vi "Configure HSDIO for Dynamic Waveform.vi"(0 "Semiconductor Module Context":T1, 1 "high level (1.8 volts)":dbl=3.3 format="%.2f", 2 "low level (0.00 volts)":dbl format="%.2f", 3 "Sample Clock Rate":dbl=104000000.0 format="%#_6p", 5 "All Pins":string[](array[string])=["CLK", "SDA", "SETID", "VIO", "HV"], 11 "error in (no error)":errorcluster) -> (15 "error out":errorcluster)   [LabVIEW 2013]
uses:
  <vilib>/NI_TestStand_SemiconductorModule/NI_TestStand_Semiconductor_Module.lvlibp/PinMap/General/SemiconductorModuleContext.ctl
  <vilib>/NI_TestStand_SemiconductorModule/NI_TestStand_Semiconductor_Module.lvlibp/PinMap/General/NIInstrumentTypeIDs.ctl
  <instrlib>/niHSDIO/niHSDIO.llb/niHSDIO_ctl Sample Clock Source Values (ComboBox).ctl
  <instrlib>/niHSDIO/niHSDIO.llb/niHSDIO_ctl Generation Mode Values (Ring).ctl
  <instrlib>/niHSDIO/niHSDIO.llb/niHSDIO_ctl Voltage Logic Family Values (Ring).ctl
  <vilib>/NI_TestStand_SemiconductorModule/NI_TestStand_Semiconductor_Module.lvlibp/PinMap/HSDIO/PinsToNIHSDIOSessions.vi
  <instrlib>/niHSDIO/niHSDIO.llb/niHSDIO Configure Data Voltage Logic Family.vi
  <instrlib>/niHSDIO/niHSDIO.llb/niHSDIO Configure Initial State (U32).vi
  <instrlib>/niHSDIO/niHSDIO.llb/niHSDIO Configure Idle State (U32).vi
  <instrlib>/niHSDIO/niHSDIO.llb/niHSDIO Configure Digital Edge Start Trigger.vi
  <vilib>/NI_TestStand_SemiconductorModule/NI_TestStand_Semiconductor_Module.lvlibp
panel:
  in  "RTD Compensation Value":i32=1 min=0 max=29
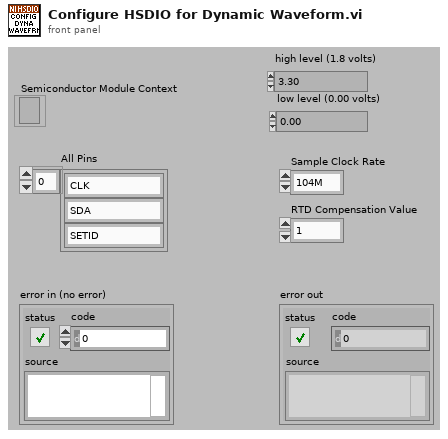
[diagram p1: front panel]
types:
  T1 = typedef "NI_TestStand_Semiconductor_Module.lvlibp/SemiconductorModuleContext.ctl" = refnum<k7>
  T2 = typedef "NI_TestStand_Semiconductor_Module.lvlibp/NIInstrumentTypeIDs.ctl" = string
  T3 = typedef "niHSDIO_ctl Voltage Logic Family Values (Ring).ctl" = i32
  T4 = typedef "niHSDIO_ctl Generation Mode Values (Ring).ctl" = i32
  T5 = typedef "niHSDIO_ctl Sample Clock Source Values (ComboBox).ctl" = string
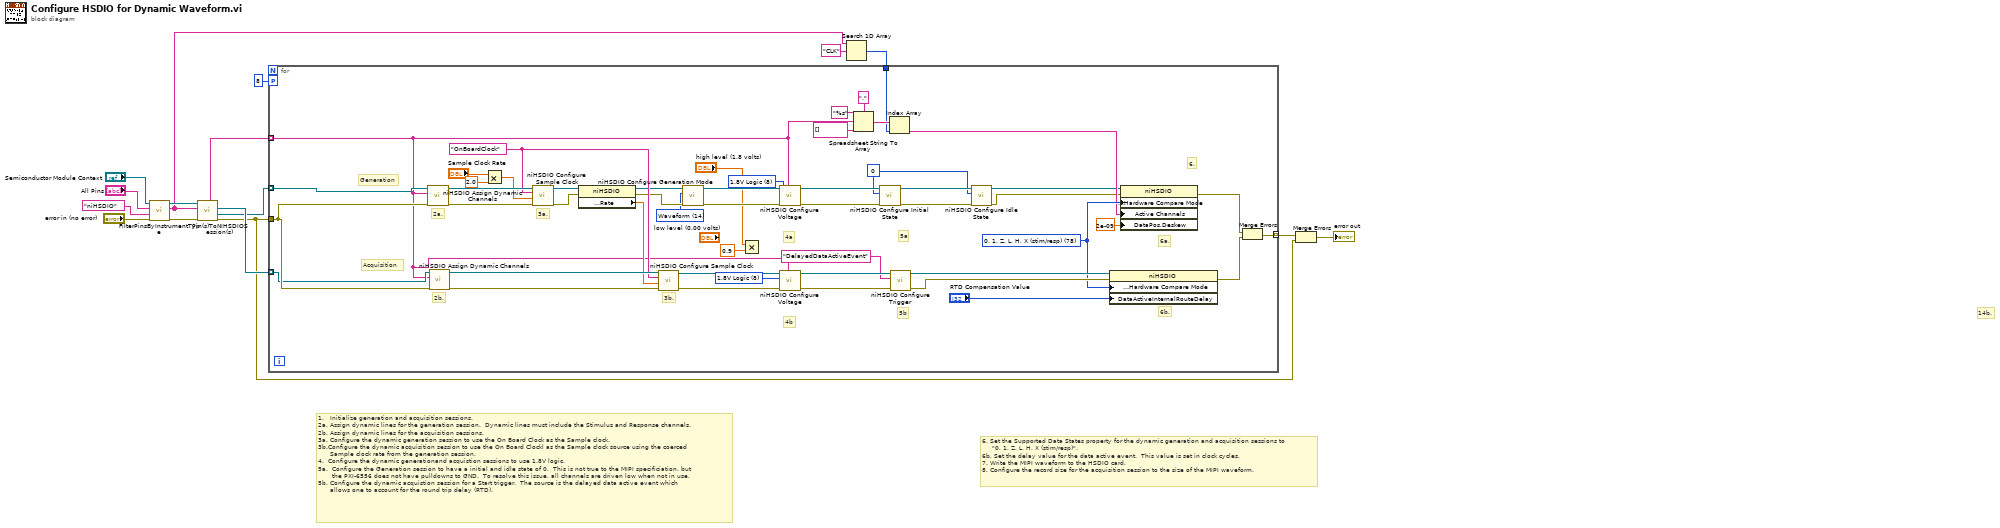
[diagram p0: block diagram]
diagram:
  # "6. Set the Supported Data States property for the dynamic generation and acquisition sessions to \n     \"0, 1, Z, L, H, X (stim/resp)\".\n6b. Set the delay value for the data active event.  This value is set in clock cycles.\n7. Write the MIPI waveform to the HSDIO card.\n8. Configure the record size for the acquisition session to the size of the MIPI waveform."
  # "1.   Initialize generation and acquisition sessions.\n2a. Assign dynamic lines for the generation session.  Dynamic lines must include the Stimulus and Response channels.\n2b. Assign dynamic lines for the acquisition sessions.\n3a. Configure the dynamic generation session to use the On Board Clock as the Sample clock.\n3b.Configure the dynamic acquisition session to use the On Board Clockl as the Sample clock source using the coerced \n      Sample clock rate from the generation session.\n4.  Configure the dynamic generationand acquistion sessions to use 1.8V logic.\n5a.  Configure the Generation session to have a initial and idle state of 0.  This is not true to the MIPI specificiation, but\n       the PXI-6556 does not have pulldowns to GND.  To resolve this issue, all channels are driven low when not in use.\n5b. Configure the dynamic acquistion session for a Start trigger.  The source is the delayed data active event which\n      allows one to account for the round trip delay (RTD)."
  # "14b."
  n1 = call <vilib>:"FilterPinsByInstrumentType.vi"("error in (no error)"="error in (no error)", "Instrument Type Id"=T2 "niHSDIO", "Pins"="All Pins", "Semiconductor Module Context"="Semiconductor Module Context") -> ("error out"=w15:errorcluster, "Filtered Pins"=w4:string[], "Semiconductor Module Context Out"=w11:T1)  [unwired: 5 in]
  n2 = call-poly <vilib>:"Pin(s)ToNIHSDIOSession(s).vi"("error in (no error)"=w15, "Pins"=w4, "Semiconductor Module Context"=w11) -> ("error out"=w6:errorcluster, "Generation Sessions"=w8:refnum<k15>[], "Acquisition Sessions"=w9:refnum<k15>[], "Channel Lists"=w2:string[])  [unwired: 3 in, 2 out]
  n3 = Search 1D Array(1D array=w4, element="CLK") -> (index of element=w1:i32)  [unwired: 1 in]
  n4 = for {
    workers-P: 8 -> [_]
    tunnel: w9 -> [w36] mode=indexing
    tunnel: w8 -> [w35] mode=indexing
    tunnel: w6 -> [w37]
    tunnel: w2 -> [w22] mode=indexing
    tunnel: [w39] -> w7 mode=indexing
    tunnel: w1 -> [w20]
    w27 = u32 0 ("initial state (0x0000)")
    w31 = T3 8 items=["5.0V Logic"=5, "3.3V Logic"=6, "2.5V Logic"=7, "1.8V Logic"=8, "1.5V Logic"=80, "1.2V Logic"=81] ("logic family (3.3V logic)")
    w32 = T3 8 items=["5.0V Logic"=5, "3.3V Logic"=6, "2.5V Logic"=7, "1.8V Logic"=8, "1.5V Logic"=80, "1.2V Logic"=81] ("logic family (3.3V logic)")
    w38 = 78 items=["0, 1 (binary)"=77, "0, 1, Z (tristate)"=83, "0, 1, Z, L, H, X (stim/resp)"=78, "L, H, X (resp only)"=79] ("Advanced:Supported Data States")
    w42 = T4 14 items=["Waveform"=14, "Scripted"=15] ("generation mode (waveform)")
    w59 = T5 "OnBoardClock" ("clock source (on board clock)")
    # "6."
    # "6b."
    # "6a."
    # "Acquisition"
    # "Generation"
    # "5a"
    # "4b"
    # "4a"
    # "5b"
    # "3b."
    # "3a."
    # "2b."
    # "2a."
    n5 = call <instrlib>:"niHSDIO Assign Dynamic Channels.vi"("error in (no error)"=w37, "channel list (all:\"\")"=w22, "instrument handle"=w35) -> ("error out"=w65:errorcluster, "instrument handle out"=w66:refnum<k15>)  [unwired: 7 in]
    n6 = call <instrlib>:"niHSDIO Assign Dynamic Channels.vi"("error in (no error)"=w37, "channel list (all:\"\")"=w22, "instrument handle"=w36) -> ("error out"=w63:errorcluster, "instrument handle out"=w64:refnum<k15>)  [unwired: 7 in]
    n7 = Multiply(x="Sample Clock Rate", y=2.0) -> (x*y=w29:dbl)
    n8 = call <instrlib>:"niHSDIO Configure Sample Clock.vi"("error in (no error)"=w65, "clock rate (50MHz)"=w29, "clock source (on board clock)"=w59, "instrument handle"=w66) -> ("error out"=w60:errorcluster, "instrument handle out"=w61:refnum<k15>)  [unwired: 6 in]
    n9 = property on="Property Node" class="niHSDIO"(reference=w61, error in=w60) -> (reference out=w44:refnum<k15>, error out=w46:errorcluster, "Timing:Sample Clock:Rate"=w62:dbl)
    n10 = call <instrlib>:"niHSDIO Configure Sample Clock.vi"("error in (no error)"=w63, "clock rate (50MHz)"=w62, "clock source (on board clock)"=w59, "instrument handle"=w64) -> ("error out"=w58:errorcluster, "instrument handle out"=w57:refnum<k15>)  [unwired: 6 in]
    n11 = call <instrlib>:"niHSDIO Configure Generation Mode.vi"("error in (no error)"=w46, "generation mode (waveform)"=w42, "instrument handle"=w44) -> ("error out"=w45:errorcluster, "instrument handle out"=w43:refnum<k15>)  [unwired: 7 in]
    n12 = Multiply(x="high level (1.8 volts)", y=0.9) -> ()  [unwired: 1 out]
    n13 = call-poly <instrlib>:"niHSDIO Configure Voltage.vi"("channel list (all:\"\")"=w22, "error in (no error)"=w45, "logic family (3.3V logic)"=w31, "instrument handle"=w43) -> ("error out"=w47:errorcluster, "instrument handle out"=w48:refnum<k15>)  [unwired: 6 in]
    n14 = call-poly <instrlib>:"niHSDIO Configure Voltage.vi"("channel list (all:\"\")"=w22, "error in (no error)"=w58, "logic family (3.3V logic)"=w32, "instrument handle"=w57) -> ("error out"=w55:errorcluster, "instrument handle out"=w56:refnum<k15>)  [unwired: 6 in]
    n15 = Spreadsheet String To Array(delimiter (Tab)=",", format string="%s", spreadsheet string=w22, array type (2D Dbl)=string[] []) -> (array=w21:string[])
    n16 = call-poly <instrlib>:"niHSDIO Configure Initial State.vi"("error in (no error)"=w47, "initial state (0x0000)"=w27, "instrument handle"=w48) -> ("error out"=w50:errorcluster, "instrument handle out"=w49:refnum<k15>)  [unwired: 7 in]
    n17 = Index Array(array=w21, index=w20) -> (element=w19:string)
    n18 = call-poly <instrlib>:"niHSDIO Configure Trigger.vi"("error in (no error)"=w55, "source (PFI 0)"="DelayedDataActiveEvent" ("channel list (all:\"\")"), "instrument handle"=w56) -> ("error out"=w51:errorcluster, "instrument handle out"=w54:refnum<k15>)  [unwired: 7 in]
    n19 = call-poly <instrlib>:"niHSDIO Configure Idle State.vi"("error in (no error)"=w50, "idle state (0x0000)"=w27, "instrument handle"=w49) -> ("error out"=w18:errorcluster, "instrument handle out"=w17:refnum<k15>)  [unwired: 7 in]
    n20 = property on="Property Node" class="niHSDIO"(reference=w54, error in=w51, "Advanced:Hardware Compare:Hardware Compare Mode"=w38, "DataActiveInternalRouteDelay"="RTD Compensation Value") -> (error out=w40:errorcluster)  [unwired: 1 out]
    n21 = property on="Property Node" class="niHSDIO"(reference=w17, error in=w18, "Advanced:Hardware Compare:Hardware Compare Mode"=w38, "Active Channels"=w19, "DataPos.Deskew"=2e-09 ("Timing:Data Position:Deskew")) -> (error out=w41:errorcluster)  [unwired: 1 out]
    n22 = Merge Errors(w41, w40) -> (w39:errorcluster)
  }
  n23 = Merge Errors(w7, w6) -> (→"error out":errorcluster)
